vi "SourceBackground.vi"(6 "首次调用？":bool, 9 "通量in":dbl[](array[numeric])) -> (0 "源与基线灯":bool, 1 "源强out":dbl[](array[numeric]), 3 "通量out":dbl[](array[numeric]))   [LabVIEW 2020]
panel:
  in  "本底减除":dbl[](array[numeric]) caption="本底减除："
  in  "通道源强":dbl[](array[numeric]) caption="通道源强："
  out "通量名称":string[](array[string]) caption="通量名称："
  in  "开关":bool caption="源与本底开关："
  in  "Tab Control":enum32{"Page 2"}(tab)
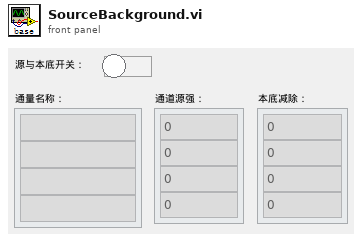
[diagram p1: front panel]
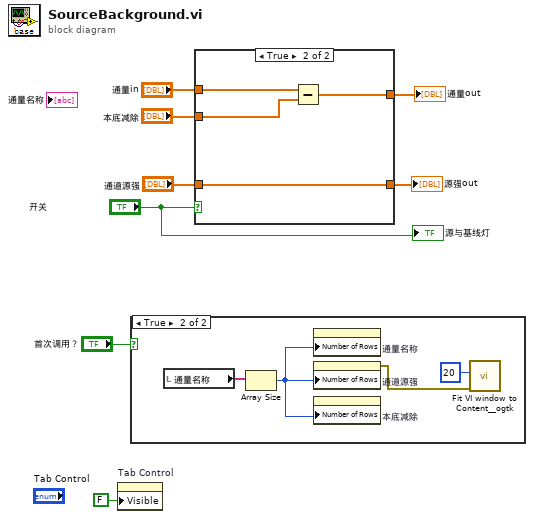
[diagram p0: block diagram]
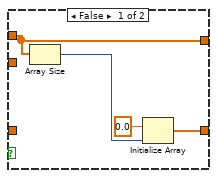
[diagram p3: hidden frame]
diagram:
  n1 = property on="Tab Control" class="TabCtl (strict)"("Visible"=FALSE) -> ()  [unwired: 2 in, 2 out]
  n2 = case shown="True" "首次调用？" {
    frame False {
    }
    frame True {
      n3 = local read "通量名称"() -> (w11:string[])
      n4 = Array Size(array=w11) -> (size(s)=w12:i32)
      n5 = property on="通量名称" class="Arr (strict)"("Number of Rows"=w12) -> ()  [unwired: 2 in, 2 out]
      n6 = property on="通道源强" class="Arr (strict)"("Number of Rows"=w12) -> (error out=w10:errorcluster)  [unwired: 2 in, 1 out]
      n7 = property on="本底减除" class="Arr (strict)"("Number of Rows"=w12) -> ()  [unwired: 2 in, 2 out]
      n8 = call <userlib>:"Fit VI window to Content__ogtk.vi"("error in (no error)"=w10, "border spacing (2 px)"=20) -> ()  [unwired: 4 in, 2 out]
    }
  }
  n9 = case shown="True" "开关" {
    tunnel: "通量in" -> [w14 w19]
    tunnel: [w14 w18] -> w3
    tunnel: "通道源强" -> [_ w20]
    tunnel: "本底减除" -> [_ w17]
    tunnel: [w15 w20] -> w6
    frame False {
      n10 = Array Size(array=w14) -> (size(s)=w13:i32)
      n11 = Initialize Array(0.0 ("元素"), w13) -> (w15:dbl[])
    }
    frame True {
      n12 = Subtract(x=w19, y=w17) -> (x-y=w18:dbl[])
    }
  }
  "通量out" <- w3
  "源强out" <- w6
  "源与基线灯" <- "开关"
